vi "4Pi Focus Lock - Norm FFT.vi"(8 "error in":errorcluster, 10 "FFT Image Dst":T1, 11 "Image In":T1) -> (0 "error out":errorcluster, 3 "FFT Image Out":T1)   [LabVIEW 2021]
uses:
  <vilib>/vision/Image Controls.llb/IMAQ Image.ctl
  <vilib>/vision/NI_Vision_Development_Module.lvlib
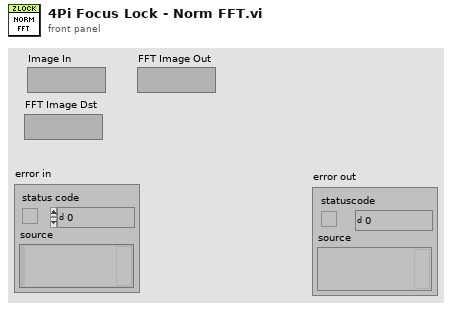
[diagram p1: front panel]
types:
  T1 = typedef "IMAQ Image.ctl" = refnum<image>
  T2 = cluster{"histogram":u32[], "Minimal Value":sgl, "Maximal Value":sgl, "Starting Value":sgl, "Interval Width":sgl, "Mean Value":sgl, "Standard  Variation":sgl, "Area (pixels)":i32}
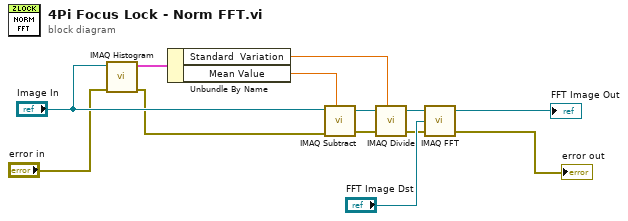
[diagram p0: block diagram]
diagram:
  n1 = call "IMAQ Histogram"("error in (no error)"="error in", "Image"="Image In") -> ("error out"=w6:errorcluster, "Histogram Report"=w13:T2)  [unwired: 8 in]
  n2 = Unbundle By Name(w13) -> ("Standard  Variation"=w11:sgl, "Mean Value"=w10:sgl)
  n3 = call "IMAQ Subtract"("Image Src A"="Image In", "Constant"=w10, "error in (no error)"=w6) -> ("Image Dst Out"=w12:T1, "error out"=w5:errorcluster)  [unwired: 4 in]
  n4 = call "IMAQ Divide"("Image Src A"=w12, "Constant"=w11, "error in (no error)"=w5) -> ("Image Dst Out"=w8:T1, "error out"=w4:errorcluster)  [unwired: 4 in]
  n5 = call "IMAQ FFT"("error in (no error)"=w4, "Image Dst"="FFT Image Dst", "Image Src"=w8) -> ("error out"=→"error out":errorcluster, "Image Dst Out"=→"FFT Image Out":T1)  [unwired: 1 in]
